vi "main.vi"() -> ()   [LabVIEW 2015]
uses:
  Stany_enum.ctl
  <vilib>/DAQmx/write.llb/DAQmx Write (Analog Wfm 1Chan NSamp).vi
  <vilib>/DAQmx/read.llb/DAQmx Read (Analog 1D DBL 1Chan NSamp).vi
  <vilib>/DAQmx/create/channels.llb/DAQmx Create Channel (AO-Voltage-Basic).vi
  <vilib>/DAQmx/configure/timing.llb/DAQmx Timing (Use Waveform).vi
  <vilib>/DAQmx/miscellaneous.llb/DAQmx Fill In Error Info.vi
  <vilib>/DAQmx/create/channels.llb/DAQmx Create Channel (AI-Voltage-Basic).vi
  <vilib>/DAQmx/configure/timing.llb/DAQmx Timing (Sample Clock).vi
  <resource>/objmgr/daqmx.rc
panel:
  in  "Sterowanie\naplikacją":cluster{"Start pomiaru":bool, "Stop":bool}
  out "Ostatni błąd":errorcluster
  in  "Ustawienia\npomiaru":T1={"Kanal pomiaru"="", "Czestotliwosc pomiaru"=1000.0, "Liczba probek na kanal pomiarowy"=1000} {"Czestotliwosc pomiaru" format="%0.2f"}
  in  "Ustawienia\ngeneratora":T2={"Kanal generatora"="", "Ksztalt sygnalu"=enum."Sine Wave", "RegenMode"=10097} {"RegenMode" items=["Allow Regeneration"=10097, "Do Not Allow Regeneration"=10158]}
  out "Generowany sygnal":waveform(dbl)(graph)
  out "Pomiar":dbl[](graph)
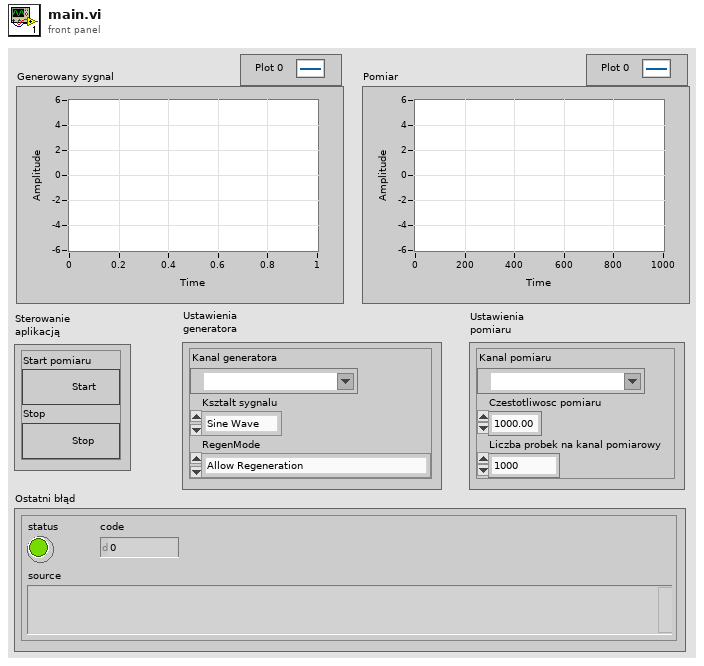
[diagram p1: front panel]
types:
  T1 = cluster{"Kanal pomiaru":tag, "Czestotliwosc pomiaru":dbl, "Liczba probek na kanal pomiarowy":i32}
  T2 = cluster{"Kanal generatora":tag, "Ksztalt sygnalu":enum16{"Sine Wave", "Triangle Wave", "Square Wave", "Sawtooth Wave"}, "RegenMode":i32}
  T3 = typedef "Stany_enum.ctl" = enum16{"Sprawdz czy STOP", "Czekaj na START", "Init", "Pracuj", "STOP", "Blad"}
  T4 = cluster{"RegenMode":refnum<vi>, "Ksztalt sygnalu":refnum<vi>, "Liczba probek na kanal pomiarowy":refnum<vi>, "Czestotliwosc pomiaru":refnum<vi>, "Kanal pomiaru":refnum<vi>, "Kanal generatora":refnum<vi>}
  T5 = enum8{"Enabled", "Disabled", "Disabled and Grayed Out"}
  T6 = enum16{"Sine Wave", "Triangle Wave", "Square Wave", "Sawtooth Wave"}
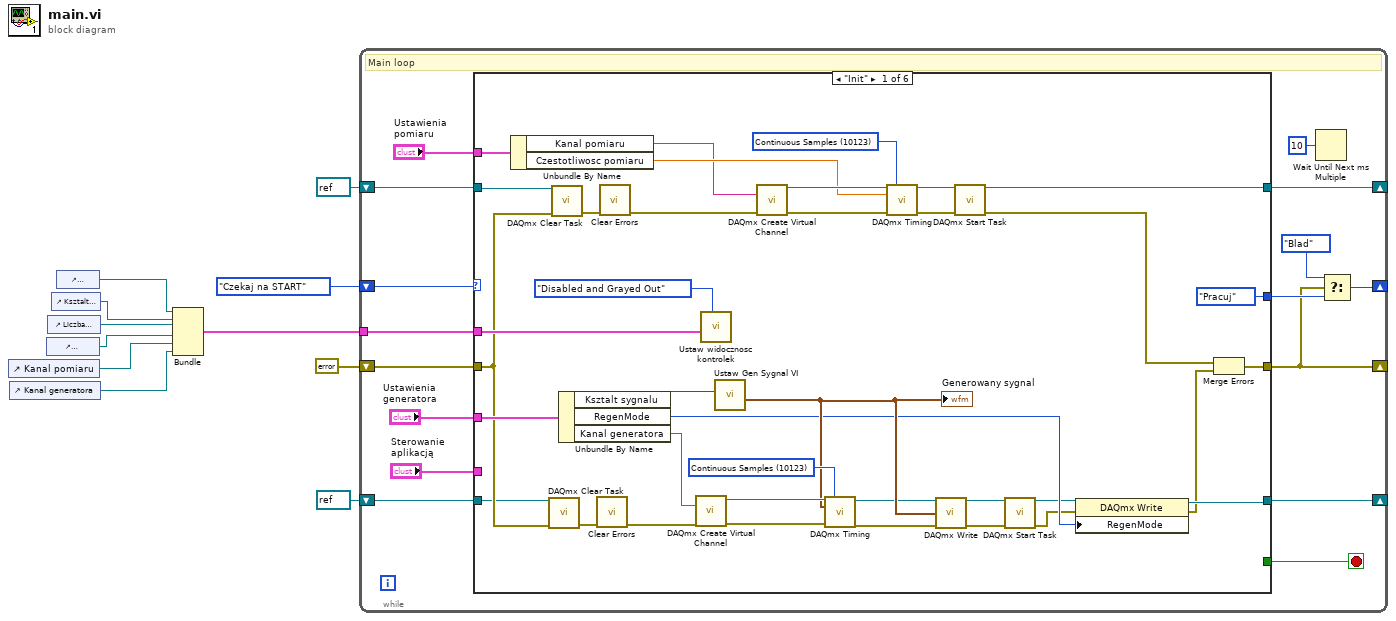
[diagram p0: block diagram]
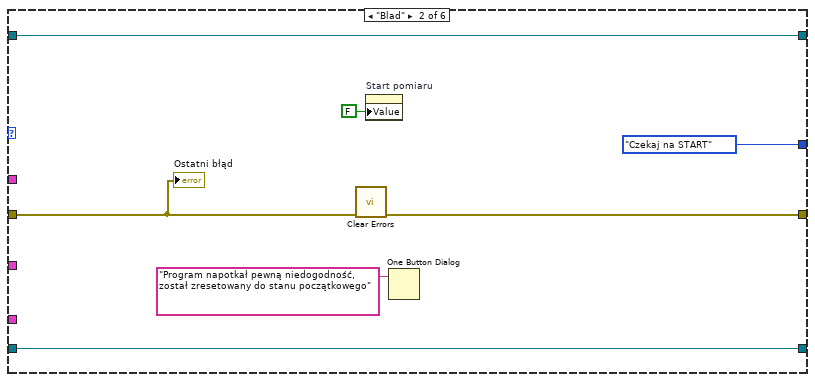
[diagram p2: hidden frame]
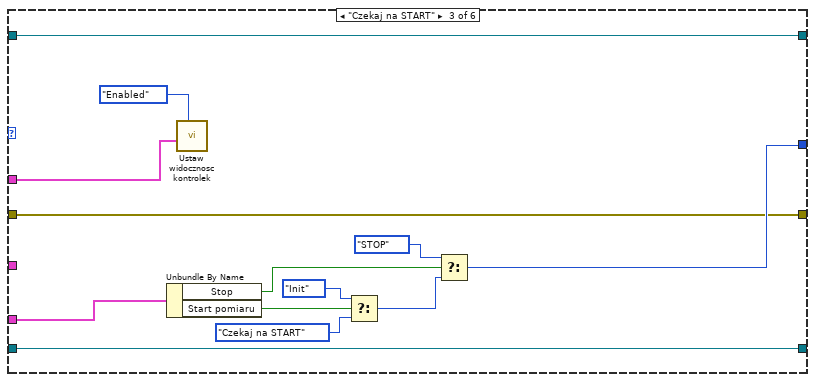
[diagram p3: hidden frame]
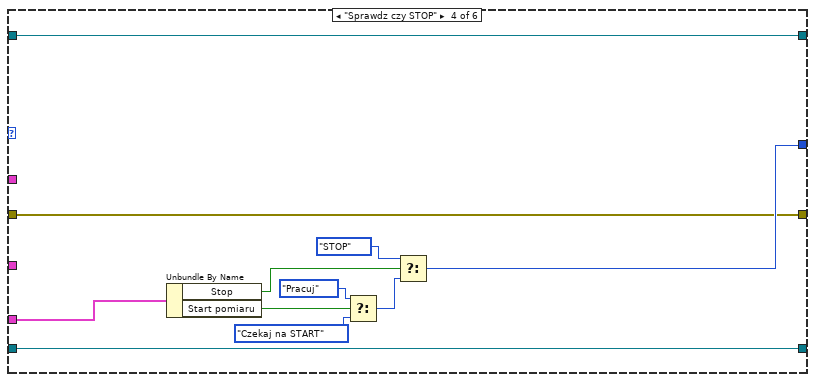
[diagram p4: hidden frame]
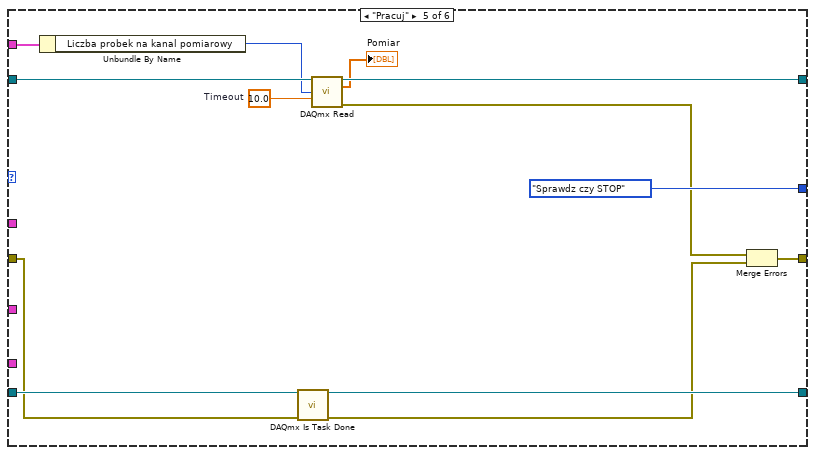
[diagram p5: hidden frame]
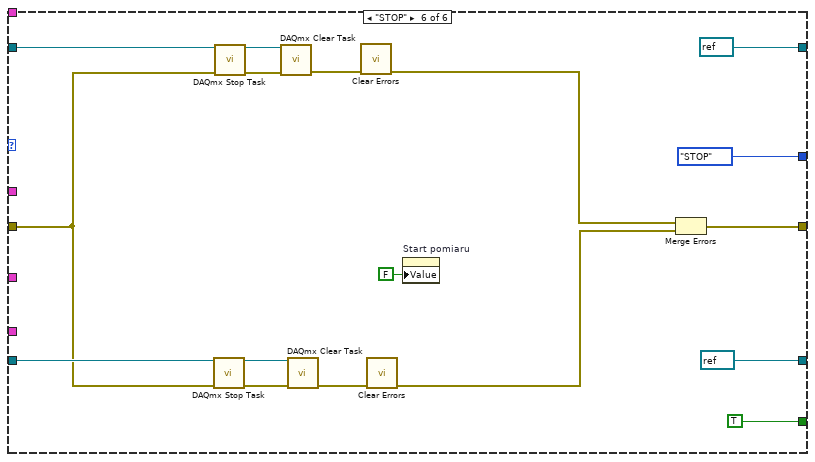
[diagram p6: hidden frame]
diagram:
  n1 = control-ref of="Kanal pomiaru"() -> (w3:refnum<vi>)
  n2 = control-ref of="Kanal generatora"() -> (w2:refnum<vi>)
  n3 = control-ref of="Czestotliwosc pomiaru"() -> (w4:refnum<vi>)
  n4 = control-ref of="Liczba probek na kanal pomiarowy"() -> (w5:refnum<vi>)
  n5 = control-ref of="Ksztalt sygnalu"() -> (w6:refnum<vi>)
  n6 = control-ref of="RegenMode"() -> (w7:refnum<vi>)
  n7 = Bundle("RegenMode"=w7, "Ksztalt sygnalu"=w6, "Liczba probek na kanal pomiarowy"=w5, "Czestotliwosc pomiaru"=w4, "Kanal pomiaru"=w3, "Kanal generatora"=w2) -> (w1:T4)  [unwired: 1 in]
  n8 = while {
    shift-right: [w26] -> _
    shift-left: refnum<k21> refnum ("task out") -> [w24]
    shift-right: [w25] -> _
    shift-left: refnum<k21> refnum ("task out") -> [w23]
    shift-right: [w17] -> _
    shift-left: Stany_enum."Czekaj na START" -> [w27]
    shift-right: [w18] -> _
    shift-left: errorcluster {"status"=FALSE, "code"=0, "source"=""} ("error out") -> [w20]
    tunnel: w1 -> [w12]
    stop <- w22 stop-if-true
    # "Main loop"
    n9 = case shown="\"Init\"" w27 {
      tunnel: [w54 w70 w79 w86 w107 refnum<k21> refnum ("task out")] -> w26
      tunnel: [w29 w71 w80 w91 w105 refnum<k21> refnum ("task out")] -> w25
      tunnel: w24 -> [w34 w70 w79 w86 w108 w119]
      tunnel: w23 -> [w32 w71 w80 w91 w106 w116]
      tunnel: [Stany_enum."Pracuj" Stany_enum."Czekaj na START" w75 w87 Stany_enum."Sprawdz czy STOP" Stany_enum."STOP"] -> w19
      tunnel: [_ _ _ _ _ TRUE] -> w22
      tunnel: "Sterowanie\naplikacją" -> [_ _ w84 w95 _ _]
      tunnel: [w47 w69 w74 w85 w100 w111] -> w18
      tunnel: w20 -> [w33 w65 w74 w85 w101 w112]
      tunnel: "Ustawienia\ngeneratora" -> [w45 _ _ _ _ _]
      tunnel: "Ustawienia\npomiaru" -> [w44 _ _ _ w97 _]
      tunnel: w12 -> [w35 _ w73 _ _ _]
      frame "Init" {
        w56 = 10123 items=["Finite Samples"=10178, "Continuous Samples"=10123, "Hardware Timed Single Point"=12522] ("sample mode")
        w62 = 10123 items=["Finite Samples"=10178, "Continuous Samples"=10123, "Hardware Timed Single Point"=12522] ("sample mode")
        n10 = Unbundle By Name(w44) -> ("Kanal pomiaru"=w42:tag, "Czestotliwosc pomiaru"=w43:dbl)
        n11 = call <vilib>:"DAQmx Clear Task.vi"("task in"=w32, "error in"=w33) -> ("error out"=w50:errorcluster)  [unwired: 13 in]
        n12 = call <vilib>:"DAQmx Clear Task.vi"("task in"=w34, "error in"=w33) -> ("error out"=w52:errorcluster)  [unwired: 13 in]
        n13 = Unbundle By Name(w45) -> ("Ksztalt sygnalu"=w38:T6, "RegenMode"=w37:i32, "Kanal generatora"=w41:tag)
        n14 = call <vilib>:"Clear Errors.vi"("error in (no error)"=w50) -> ("error out"=w49:errorcluster)  [unwired: 5 in, 1 out]
        n15 = call <vilib>:"Clear Errors.vi"("error in (no error)"=w52) -> ("error out"=w51:errorcluster)  [unwired: 5 in, 1 out]
        n16 = call-poly <vilib>:"DAQmx Create Virtual Channel.vi"("physical channels"=w41, "error in"=w49) -> ("task out"=w55:refnum<k21>, "error out"=w57:errorcluster)  [unwired: 12 in]
        n17 = call "Ustaw widocznosc kontrolek.vi"("Disabled/Enabled"=T5."Disabled and Grayed Out" ("Disabled"), "Klaster referencji"=w35) -> ()  [unwired: 10 in]
        n18 = call "Ustaw Gen Sygnal VI.vi"("Ksztalt sygnalu"=w38) -> ("generowany sygnal"=w46:waveform(dbl))  [unwired: 10 in]
        "Generowany sygnal" <- w46
        n19 = call-poly <vilib>:"DAQmx Create Virtual Channel.vi"("physical channels"=w42, "error in"=w51) -> ("task out"=w63:refnum<k21>, "error out"=w64:errorcluster)  [unwired: 12 in]
        n20 = call-poly <vilib>:"DAQmx Timing.vi"("task/channels in"=w55, "sample mode"=w56, "waveform"=w46, "error in"=w57) -> ("task out"=w39:refnum<k21>, "error out"=w58:errorcluster)  [unwired: 10 in]
        n21 = call-poly <vilib>:"DAQmx Timing.vi"("task/channels in"=w63, "sample mode"=w62, "rate"=w43, "error in"=w64) -> ("task out"=w40:refnum<k21>, "error out"=w61:errorcluster)  [unwired: 10 in]
        n22 = call-poly <vilib>:"DAQmx Write.vi"("task/channels in"=w39, "data"=w46, "error in"=w58) -> ("task out"=w60:refnum<k21>, "error out"=w59:errorcluster)  [unwired: 10 in, 1 out]
        n23 = call <vilib>:"DAQmx Start Task.vi"("task/channels in"=w40, "error in"=w61) -> ("task out"=w54:refnum<k21>, "error out"=w48:errorcluster)  [unwired: 12 in]
        n24 = call <vilib>:"DAQmx Start Task.vi"("task/channels in"=w60, "error in"=w59) -> ("task out"=w31:refnum<k21>, "error out"=w30:errorcluster)  [unwired: 12 in]
        n25 = property class="DAQmx Write"(reference=w31, error in=w30, "RegenMode"=w37) -> (reference out=w29:refnum<k21>, error out=w28:errorcluster)
        n26 = Merge Errors(w48, w28) -> (w47:errorcluster)
      }
      frame "Blad" {
        n27 = call <vilib>:"Clear Errors.vi"("error in (no error)"=w65) -> ("error out"=w69:errorcluster)  [unwired: 5 in, 1 out]
        n28 = property on="Start pomiaru" class="Bool (strict)"("Value"=FALSE) -> ()  [unwired: 2 in, 2 out]
        n29 = One Button Dialog(message="Program napotkał pewną niedogodność, został zresetowany do stanu początkowego") -> ()  [unwired: 1 in, 1 out]
        "Ostatni błąd" <- w65
      }
      frame "Czekaj na START" {
        n30 = Unbundle By Name(w84) -> ("Stop"=w78:bool, "Start pomiaru"=w83:bool)
        n31 = call "Ustaw widocznosc kontrolek.vi"("Disabled/Enabled"=T5."Enabled", "Klaster referencji"=w73) -> ()  [unwired: 10 in]
        n32 = Select(t=Stany_enum."Init", s=w83, f=Stany_enum."Czekaj na START") -> (s? t:f=w77:T3)
        n33 = Select(t=Stany_enum."STOP", s=w78, f=w77) -> (s? t:f=w75:T3)
      }
      frame "Sprawdz czy STOP" {
        n34 = Unbundle By Name(w95) -> ("Stop"=w90:bool, "Start pomiaru"=w94:bool)
        n35 = Select(t=Stany_enum."Pracuj", s=w94, f=Stany_enum."Czekaj na START") -> (s? t:f=w88:T3)
        n36 = Select(t=Stany_enum."STOP", s=w90, f=w88) -> (s? t:f=w87:T3)
      }
      frame "Pracuj" {
        w104 = 10.0  # Timeout
        n37 = Unbundle By Name(w97) -> ("Liczba probek na kanal pomiarowy"=w96:i32)
        n38 = call <vilib>:"DAQmx Is Task Done.vi"("task/channels in"=w106, "error in"=w101) -> ("task out"=w105:refnum<k21>, "error out"=w98:errorcluster)  [unwired: 11 in, 1 out]
        n39 = call-poly <vilib>:"DAQmx Read.vi"("task/channels in"=w108, "number of samples per channel"=w96, "timeout"=w104) -> ("task out"=w107:refnum<k21>, "data"=→"Pomiar":dbl[], "error out"=w99:errorcluster)  [unwired: 10 in]
        n40 = Merge Errors(w99, w98) -> (w100:errorcluster)
      }
      frame "STOP" {
        n41 = call <vilib>:"DAQmx Stop Task.vi"("task/channels in"=w116, "error in"=w112) -> ("task out"=w117:refnum<k21>, "error out"=w118:errorcluster)  [unwired: 12 in]
        n42 = call <vilib>:"DAQmx Stop Task.vi"("task/channels in"=w119, "error in"=w112) -> ("task out"=w121:refnum<k21>, "error out"=w120:errorcluster)  [unwired: 12 in]
        n43 = call <vilib>:"DAQmx Clear Task.vi"("task in"=w121, "error in"=w120) -> ("error out"=w114:errorcluster)  [unwired: 13 in]
        n44 = call <vilib>:"DAQmx Clear Task.vi"("task in"=w117, "error in"=w118) -> ("error out"=w113:errorcluster)  [unwired: 13 in]
        n45 = call <vilib>:"Clear Errors.vi"("error in (no error)"=w114) -> ("error out"=w110:errorcluster)  [unwired: 5 in, 1 out]
        n46 = call <vilib>:"Clear Errors.vi"("error in (no error)"=w113) -> ("error out"=w109:errorcluster)  [unwired: 5 in, 1 out]
        n47 = property on="Start pomiaru" class="Bool (strict)"("Value"=FALSE ("Start pomiaru")) -> ()  [unwired: 2 in, 2 out]
        n48 = Merge Errors(w110, w109) -> (w111:errorcluster)
      }
    }
    n49 = Wait Until Next ms Multiple(millisecond multiple=u32 10) -> ()  [unwired: 1 out]
    n50 = Select(t=Stany_enum."Blad", s=w18, f=w19) -> (s? t:f=w17:T3)
  }
